vi "写.vi"(8 "error in (no error)":errorcluster caption="错误输入（无错误）", 10 "写入缓冲区":string, 11 "通讯 输入":refnum<class "通讯.lvclass">) -> (0 "error out":errorcluster caption="错误输出", 3 "通讯 输出":refnum<class "通讯.lvclass">)   [LabVIEW 2015, in "通讯.lvlib" / "通讯.lvclass"]
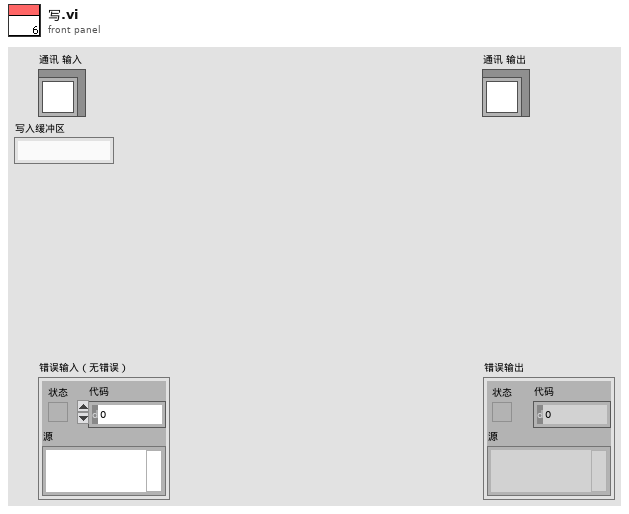
[diagram p1: front panel]
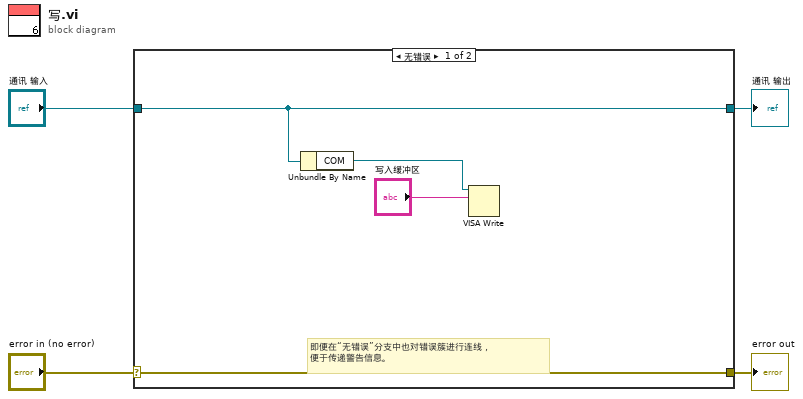
[diagram p0: block diagram]
diagram:
  n1 = case shown="无错误" "error in (no error)" {
    selector: "error in (no error)" -> [w8 w10]
    tunnel: [w8 w10] -> w3
    tunnel: [w7 w9] -> w1
    tunnel: "通讯 输入" -> [w7 w9]
    frame No Error {
      # "即便在“无错误”分支中也对错误簇进行连线，\n便于传递警告信息。"
      n2 = Unbundle By Name(w7) -> ("COM"=w6:refnum<visa-resource-name>)
      n3 = VISA Write(VISA resource name=w6, write buffer="写入缓冲区") -> ()  [unwired: 1 in, 3 out]
    }
    frame Error {
    }
  }
  "error out" <- w3
  "通讯 输出" <- w1
